vi "Update Title.vi"(8 "error in (no error)":errorcluster, 10 "title":string, 11 "[V] Waveform in":refnum<class "[V] Waveform.lvclass">) -> (0 "error out":errorcluster, 3 "[V] Waveform out":refnum<class "[V] Waveform.lvclass">)   [LabVIEW 2020, in "[V] Waveform.lvlib" / "[V] Waveform.lvclass"]
uses:
  [V] Waveform.lvclass
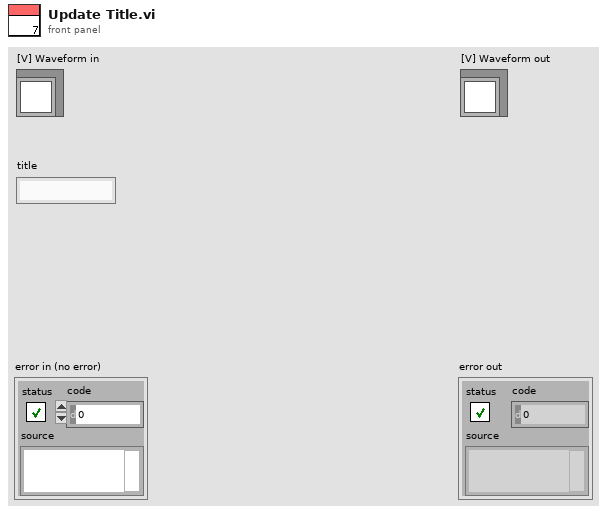
[diagram p1: front panel]
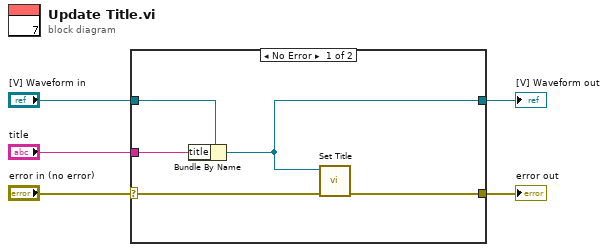
[diagram p0: block diagram]
diagram:
  n1 = case shown="No Error" "error in (no error)" {
    selector: "error in (no error)" -> [w10 w12]
    tunnel: [w9 w12] -> w4
    tunnel: [w6 w11] -> w2
    tunnel: "[V] Waveform in" -> [w8 w11]
    tunnel: "title" -> [w7 _]
    frame No Error {
      n2 = Bundle By Name(cluster=w8, "title"=w7) -> (w6:refnum<class "[V] Waveform.lvclass">)
      n3 = call "Set Title.vi"("error in (no error)"=w10, "[V] Waveform in"=w6) -> ("error out"=w9:errorcluster)  [unwired: 8 in, 1 out]
    }
    frame Error {
    }
  }
  "error out" <- w4
  "[V] Waveform out" <- w2
